vi "InitConnection.vi"(8 "error in (no error)":errorcluster, 11 "Acquisition in":refnum<class "Acquisition.lvclass">) -> (0 "error out":errorcluster, 3 "Acquisition out":refnum<class "Acquisition.lvclass">)   [LabVIEW 2018, in "Acquisition.lvclass"]
uses:
  Acquisition.lvclass
  Server/Server.lvclass
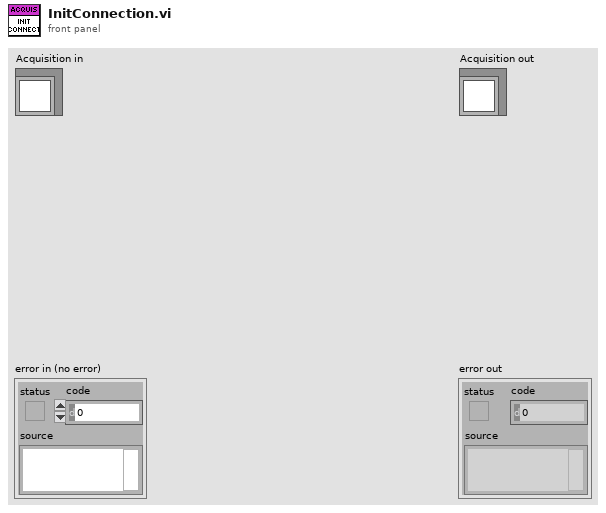
[diagram p1: front panel]
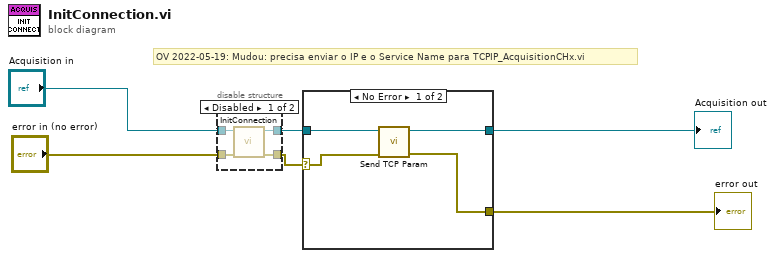
[diagram p0: block diagram]
diagram:
  # "OV 2022-05-19: Mudou: precisa enviar o IP e o Service Name para TCPIP_AcquisitionCHx.vi"
  n1 = disable-structure shown="Disabled" {
    disable-tunnel: "error in (no error)" -> [w10 w11]
    disable-tunnel: "Acquisition in" -> [w9 w12]
    disable-tunnel: [w8 w12] -> w6
    disable-tunnel: [w7 w11] -> w5
    frame Disabled {
      n2 = call-parent "InitConnection.vi"("error in (no error)"=w10, "Server in"=w9) -> ("error out"=w7:errorcluster, "Server out"=w8:refnum<class "Acquisition.lvclass">)  [unwired: 8 in]
    }
    frame Enabled {
    }
  }
  n3 = case shown="No Error" w5 {
    selector: w5 -> [w15 w17]
    tunnel: w6 -> [w16 w18]
    tunnel: [w14 w17] -> w1
    tunnel: [w13 w18] -> w4
    frame No Error {
      n4 = call-dynamic "Send TCP Param.vi"("error in (no error)"=w15, "Server in"=w16) -> ("error out"=w14:errorcluster, "Server out"=w13:refnum<class "Acquisition.lvclass">)  [unwired: 8 in]
    }
    frame Error {
    }
  }
  "error out" <- w1
  "Acquisition out" <- w4
